vi "CRYPut To Curve Library.vi"(4 "O_Signal Type In":string[][](array[string]), 6 "I_Signal Type In":string[][](array[string]), 8 "O_Calibrated Device Name In":string[][](array[string]), 9 "I_Calibrated Device Name In":string[][](array[string]), 10 "Hardware In":string, 11 "Calibration Step Cluster":T3 {"Calibration 2D"."Sens Curve"."Z data" items=["dB", "Lin"]; "Calibration 2D"."Sens Curve"."X data" items=["dB", "Lin"]; "Calibration 2D"."Sens Curve"."Y data" items=["dB", "Lin"]; "Calibration 2D"."Sens Curve"."Z dB ref" format="%.1f"; "Calibration 2D"."Sens Curve"."Z axis" items=["Log", "Lin"]; "Calibration 2D"."Sens Curve"."X dB ref" format="%.1f"; "Calibration 2D"."Sens Curve"."X axis" items=["Log", "Lin"]; "Calibration 2D"."Sens Curve"."Y axis" items=["Log", "Lin"]; "Calibration 2D"."Sens Curve"."Y dB ref" format="%.1f"; "Calibration 2D"."Sens Curve"."Curve"."z" format="%.2f"; "Calibration 2D"."Sens Curve"."Curve"."y" format="%.2f"; "Calibration 2D"."Sens Curve"."Curve"."x" format="%.2f"; "Calibration 2D"."EQ Curve"."Z data" items=["dB", "Lin"]; "Calibration 2D"."EQ Curve"."X data" items=["dB", "Lin"]; "Calibration 2D"."EQ Curve"."Y data" items=["dB", "Lin"]; "Calibration 2D"."EQ Curve"."Z dB ref" format="%.1f"; "Calibration 2D"."EQ Curve"."Z axis" items=["Log", "Lin"]; "Calibration 2D"."EQ Curve"."X dB ref" format="%.1f"; "Calibration 2D"."EQ Curve"."X axis" items=["Log", "Lin"]; "Calibration 2D"."EQ Curve"."Y axis" items=["Log", "Lin"]; "Calibration 2D"."EQ Curve"."Y dB ref" format="%.1f"; "Calibration 2D"."EQ Curve"."Curve"."z" format="%.2f"; "Calibration 2D"."EQ Curve"."Curve"."y" format="%.2f"; "Calibration 2D"."EQ Curve"."Curve"."x" format="%.2f"; "Calibration 2D"."Corr Curve"."Z data" items=["dB", "Lin"]; "Calibration 2D"."Corr Curve"."X data" items=["dB", "Lin"]; "Calibration 2D"."Corr Curve"."Y data" items=["dB", "Lin"]; "Calibration 2D"."Corr Curve"."Z dB ref" format="%.1f"; "Calibration 2D"."Corr Curve"."Z axis" items=["Log", "Lin"]; "Calibration 2D"."Corr Curve"."X dB ref" format="%.1f"; "Calibration 2D"."Corr Curve"."X axis" items=["Log", "Lin"]; "Calibration 2D"."Corr Curve"."Y axis" items=["Log", "Lin"]; "Calibration 2D"."Corr Curve"."Y dB ref" format="%.1f"; "Calibration 2D"."Corr Curve"."Curve"."z" format="%.2f"; "Calibration 2D"."Corr Curve"."Curve"."y" format="%.2f"; "Calibration 2D"."Corr Curve"."Curve"."x" format="%.2f"; "Calibration 2D"."Calibration"."EQ Step size" items=["R10", "R20", "R40", "R80", "User"]; "Calibration 2D"."Calibration"."Corr Step size" items=["R10", "R20", "R40", "R80", "User"]}) -> (3 "Calibration flattened":string)   [LabVIEW 2013]
uses:
  Typedef Control/CRYCalibration All Cluster.ctl
  Typedef Control/CRYCalibration 2DCluster.ctl
  Typedef Control/CRYCalibration Cluster.ctl
  Typedef Control/CRYData Cluster.ctl
  Typedef Control/CRYData Cluster Array.ctl
  CRYProject/CRYProject Editor Global.vi
panel:
  out "Array":string[](array[string])
  out "Curve State":string[][](array[string])
  out "Values":T1 {"Z data" items=["dB", "Lin"]; "X data" items=["dB", "Lin"]; "Y data" items=["dB", "Lin"]; "Z dB ref" format="%.1f"; "Z axis" items=["Log", "Lin"]; "X dB ref" format="%.1f"; "X axis" items=["Log", "Lin"]; "Y axis" items=["Log", "Lin"]; "Y dB ref" format="%.1f"; "Curve"."z" format="%.2f"; "Curve"."y" format="%.2f"; "Curve"."x" format="%.2f"}
  out "Curve array":T1 {"Z data" items=["dB", "Lin"]; "X data" items=["dB", "Lin"]; "Y data" items=["dB", "Lin"]; "Z dB ref" format="%.1f"; "Z axis" items=["Log", "Lin"]; "X dB ref" format="%.1f"; "X axis" items=["Log", "Lin"]; "Y axis" items=["Log", "Lin"]; "Y dB ref" format="%.1f"; "Curve"."z" format="%.2f"; "Curve"."y" format="%.2f"; "Curve"."x" format="%.2f"}
  # "Insert Calibration curve and value into Curves Library"
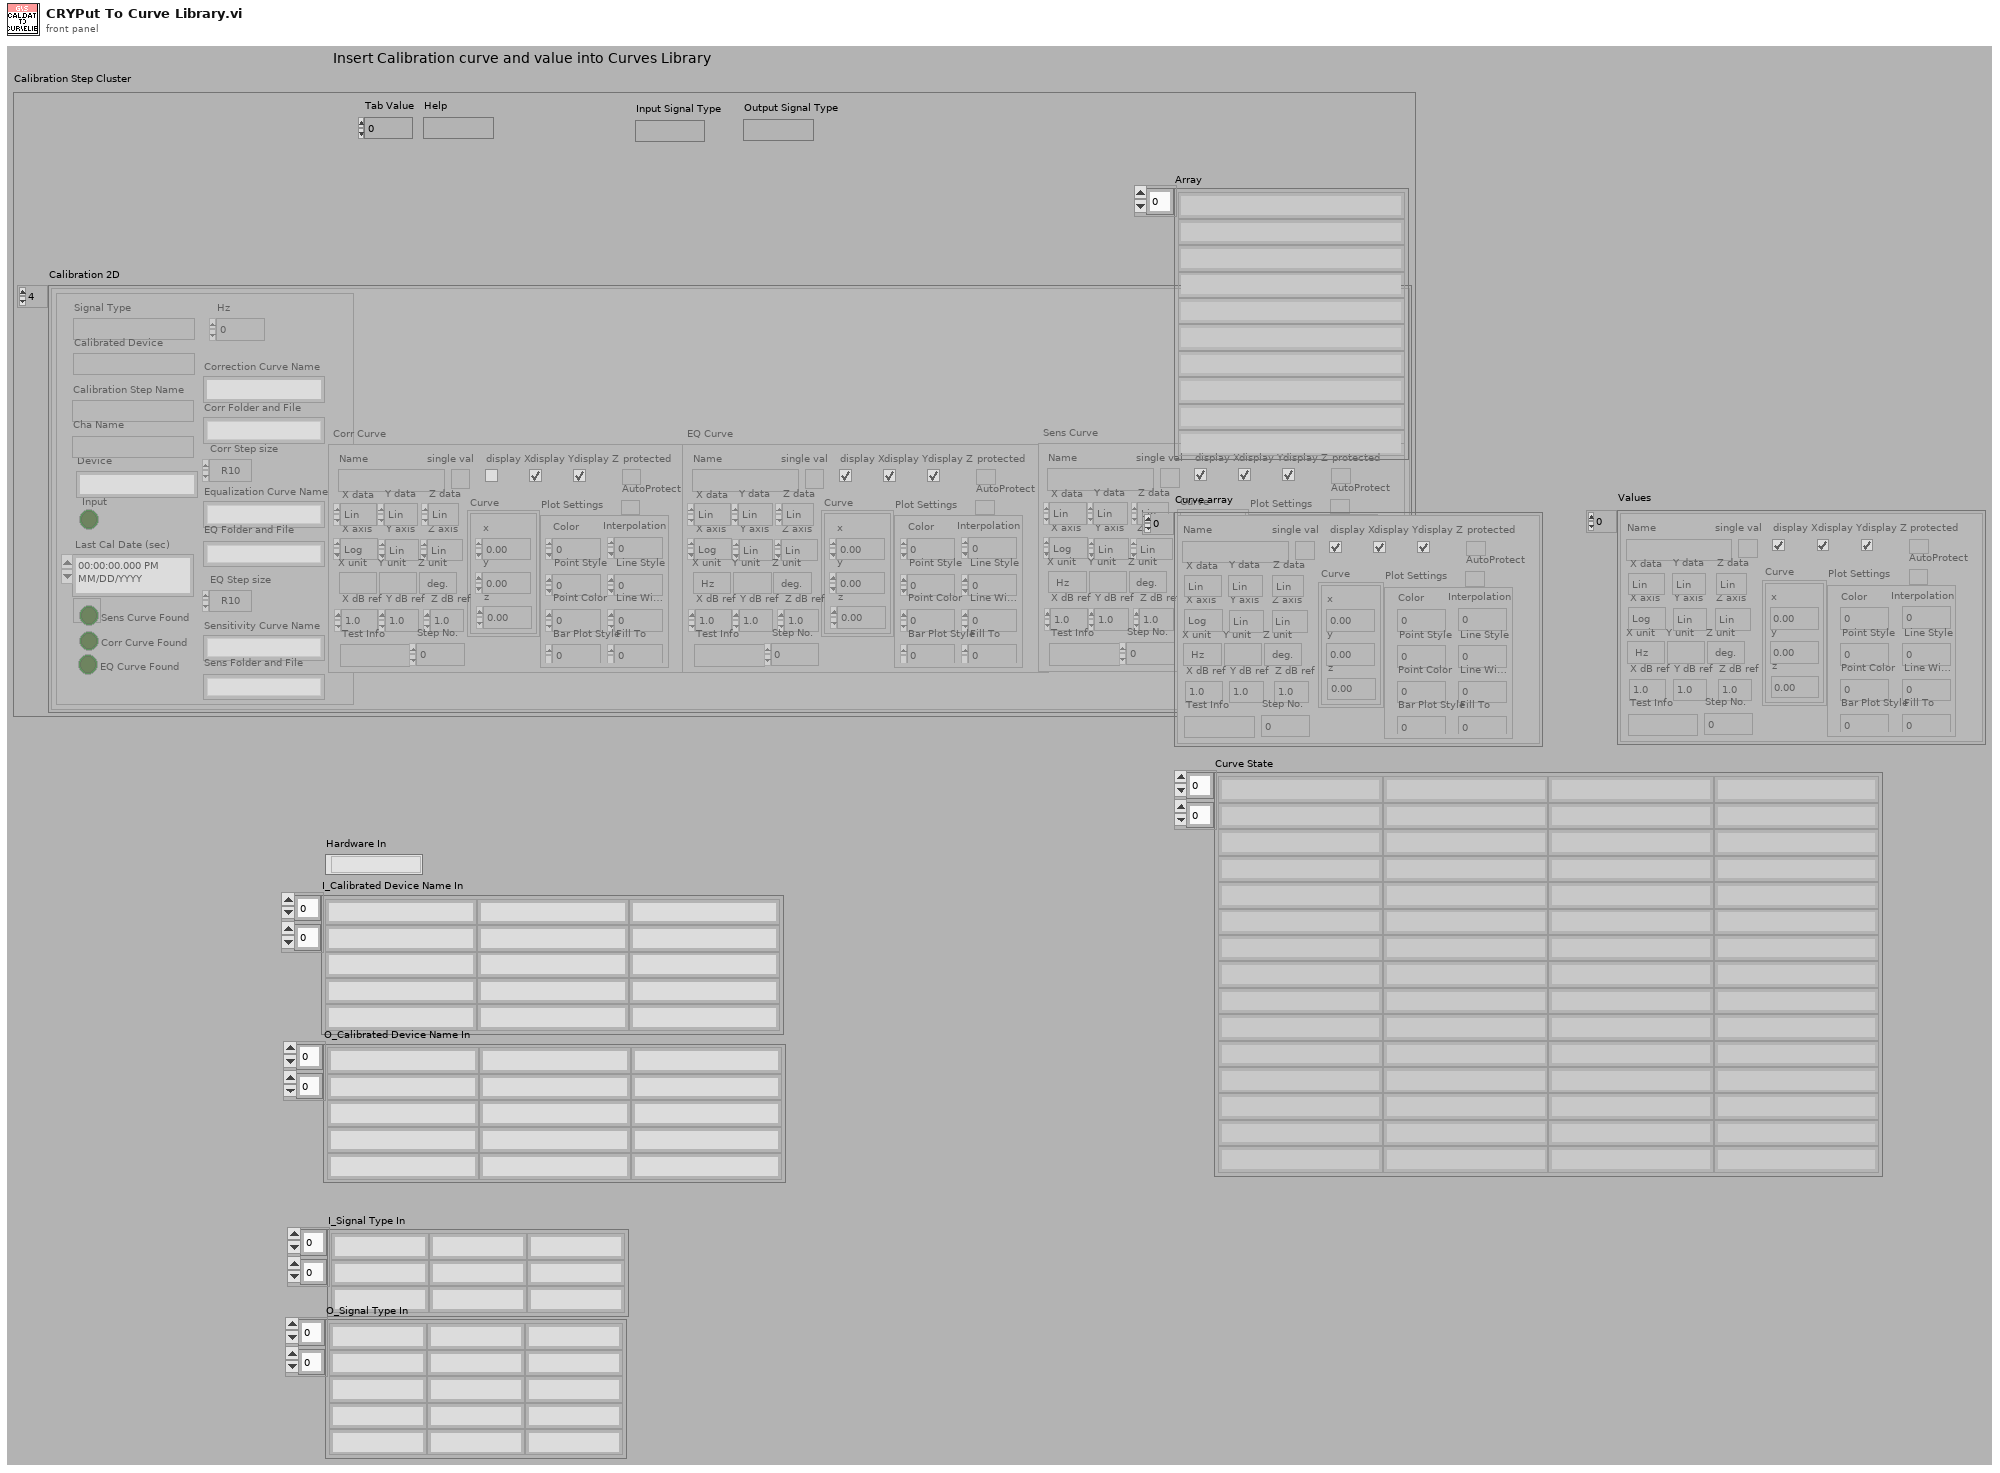
[diagram p1: front panel]
types:
  T1 = typedef "CRYData Cluster Array.ctl" = T2[]
  T2 = typedef "CRYData Cluster.ctl" = cluster{"Name":string, "Curve":cluster{"x":dbl, "y":dbl, "z":dbl}[], "X data":u16, "Y data":u16, "Z data":u16, "X axis":u16, "Y axis":u16, "Z axis":u16, "X unit":string, "Y unit":string, "Z unit":string, "X dB ref":dbl, "Y dB ref":dbl, "Z dB ref":dbl, "single val":bool, "protected":bool, "display X":bool, "display Y":bool, "display Z":bool, "Test Info":string, "Step No.":i32, "Plot Settings":cluster{"Color":u32, "Interpolation":u8, "Point Style":u8, "Line Style":u8, "Point Color":u32, "Line Width":u8, "Bar Plot Style":u8, "Fill To":i16}, "AutoProtect":bool}
  T3 = typedef "CRYCalibration All Cluster.ctl" = cluster{"Calibration 2D":T4[], "Help":string, "Tab Value":i32, "Input Signal Type":string, "Output Signal Type":string}
  T4 = typedef "CRYCalibration 2DCluster.ctl" = cluster{"Calibration":T5, "Corr Curve":T2, "EQ Curve":T2, "Sens Curve":T2}
  T5 = typedef "CRYCalibration Cluster.ctl" = cluster{"Calibration Step Name":string, "Device":string, "Correction Curve Name":string, "Equalization Curve Name":string, "Sensitivity Curve Name":string, "Corr Folder and File":string, "EQ Folder and File":string, "Sens Folder and File":string, "Corr Step size":u16, "EQ Step size":u16, "Input":bool, "Last Cal Date (sec)":timestamp, "Cha Name":string, "Corr Curve Found":bool, "EQ Curve Found":bool, "Sens Curve Found":bool, "Signal Type":string, "Calibrated Device":string, "Hz":u32}
  T6 = typedef "CRYChanged Names Cluster.ctl" = cluster{"Input Channel":T7, "Output Channel":T7, "Cuve":T7, "Value":T7, "Result":T7, "Wave":T7}
  T7 = typedef "CRYChanged Data Array Cluster.ctl" = cluster{"Rename":T8[], "Delete":T8[]}
  T8 = typedef "CRYChanged Data Cluster.ctl" = cluster{"Old Name":string, "New Name":string}
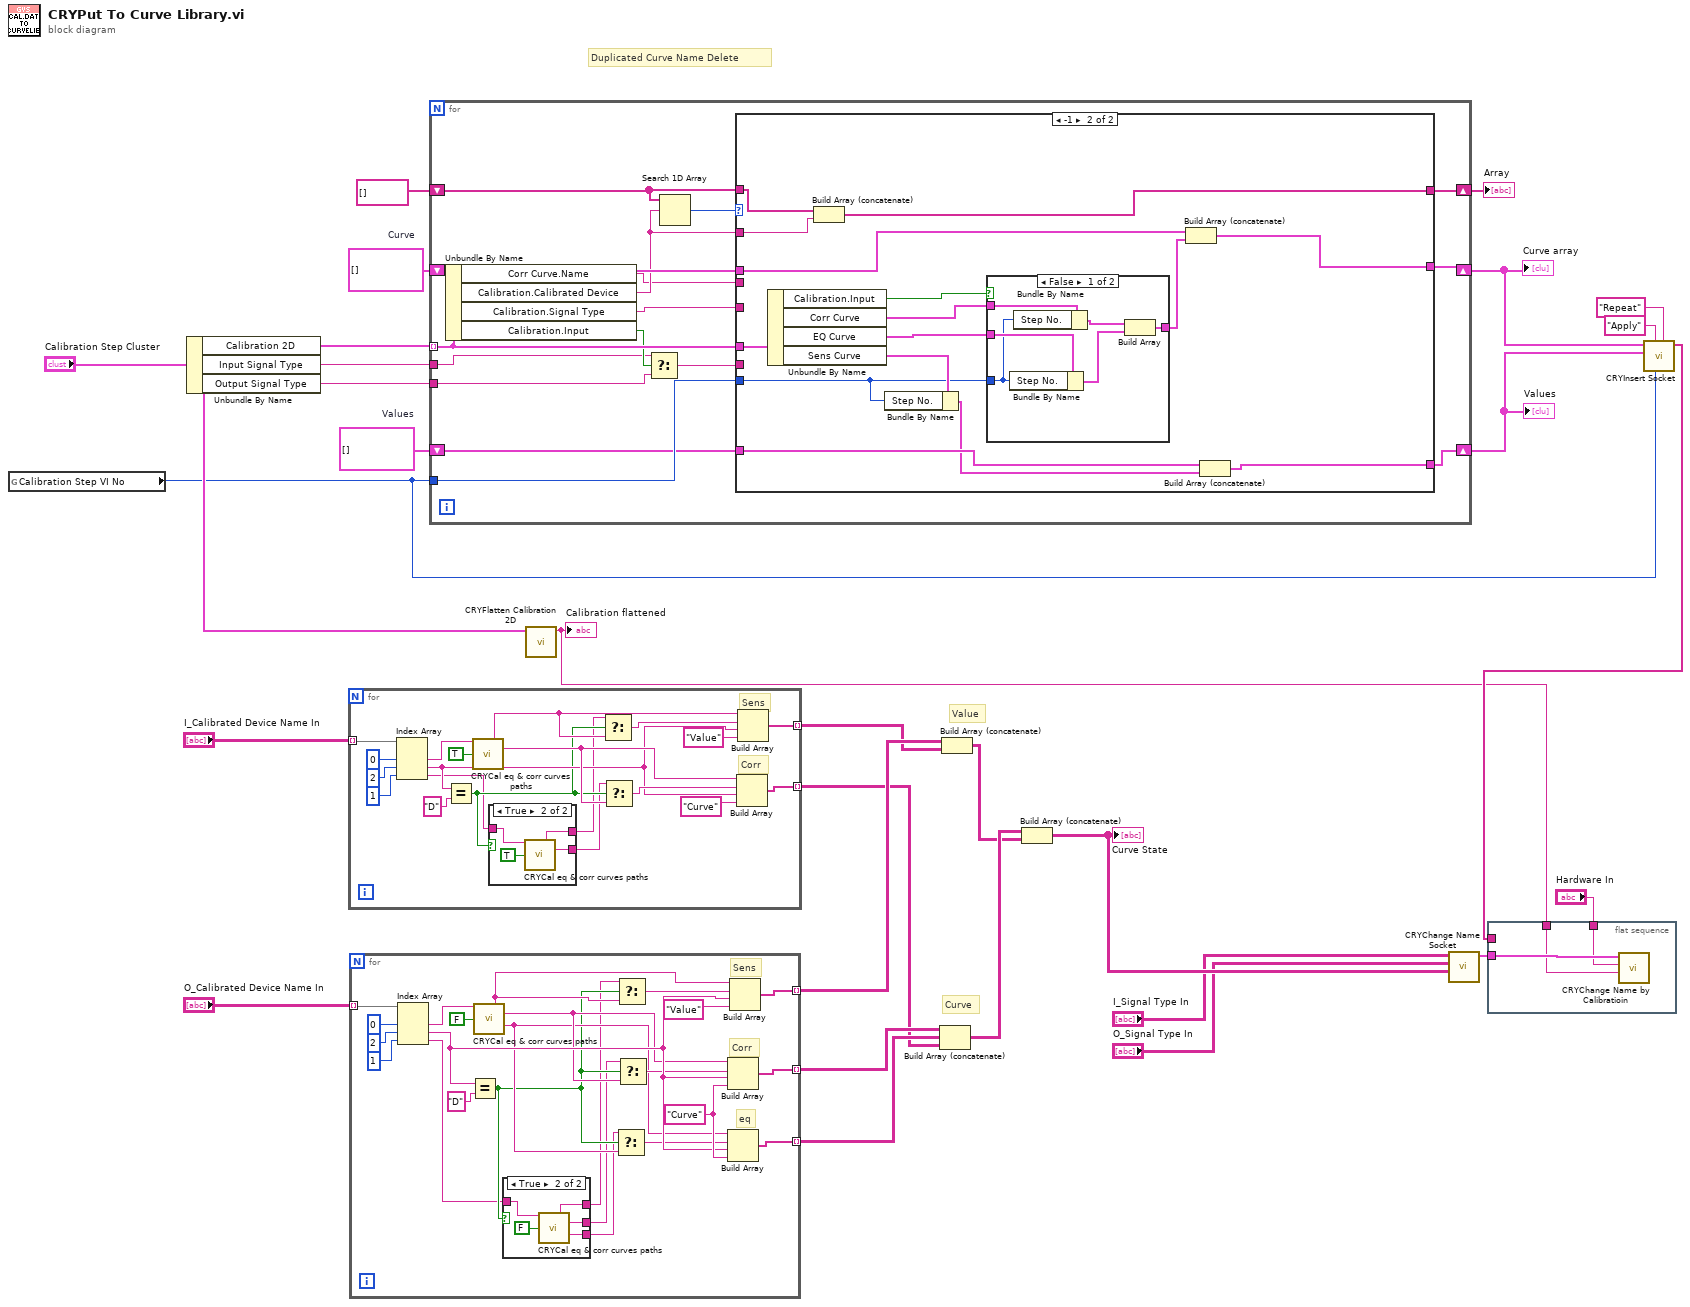
[diagram p0: block diagram]
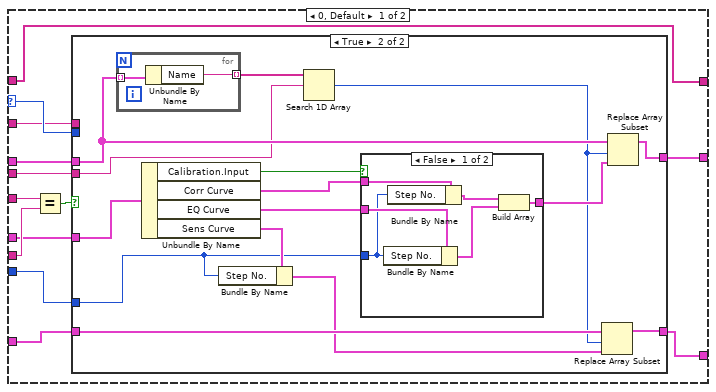
[diagram p4: hidden frame]
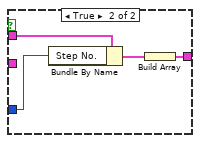
[diagram p6: hidden frame]
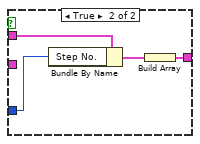
[diagram p7: hidden frame]
diagram:
  w21 = T1 []  # Values
  w25 = T1 []  # Curve
  # "Curve"
  # "Value"
  # "Duplicated Curve Name Delete"
  n1 = global read "CRYProject Editor Global.vi" "Calibration Step VI No"() -> (w24:i32)
  n2 = Unbundle By Name("Calibration Step Cluster") -> ("Calibration 2D"=w27:T4[], "Input Signal Type"=w3:string, "Output Signal Type"=w2:string)
  n3 = for {
    tunnel: "I_Calibrated Device Name In" -> [w49] mode=indexing
    tunnel: [w44] -> w16 mode=indexing
    tunnel: [w43] -> w13 mode=indexing
    # "Corr"
    # "Sens"
    n4 = Index Array(array=w49, index #1=0 ("index"), index #2=2 ("index"), index #3=1 ("index")) -> (element #1=w48:string, element #2=w36:string, element #3=w32:string)
    n5 = Equal?(x=w36, y="D" ("element")) -> (x = y?=w33:bool)
    n6 = call "CRYCal eq & corr curves paths.vi"("Calibrated Device Name"=w48, "In_Out"=TRUE) -> ("Sens Currve Name"=w35:string, "Corr Curve Name"=w39:string)  [unwired: 1 in, 11 out]
    n7 = case shown="True" w33 {
      tunnel: w32 -> [_ w52]
      tunnel: [_ w51] -> w31
      tunnel: [_ w50] -> w30
      frame False {
      }
      frame True {
        n8 = call "CRYCal eq & corr curves paths.vi"("Calibrated Device Name"=w52, "In_Out"=TRUE) -> ("Sens Currve Name"=w51:string, "Corr Curve Name"=w50:string)  [unwired: 1 in, 11 out]
      }
    }
    n9 = Select(t=w31, s=w33, f=w35) -> (s? t:f=w34:string)
    n10 = Select(t=w30, s=w33, f=w39) -> (s? t:f=w37:string)
    n11 = Build Array(w39, w37, w36, "Curve" ("element")) -> (w43:string[])
    n12 = Build Array(w35, w34, w36, "Value" ("element")) -> (w44:string[])
  }
  n13 = for {
    tunnel: "O_Calibrated Device Name In" -> [w77] mode=indexing
    tunnel: [w72] -> w17 mode=indexing
    tunnel: [w71] -> w15 mode=indexing
    tunnel: [w70] -> w14 mode=indexing
    w69 = "Curve" ("element")
    # "eq"
    # "Corr"
    # "Sens"
    n14 = Index Array(array=w77, index #1=0 ("index"), index #2=2 ("index"), index #3=1 ("index")) -> (element #1=w76:string, element #2=w66:string, element #3=w57:string)
    n15 = Equal?(x=w66, y="D" ("element")) -> (x = y?=w58:bool)
    n16 = call "CRYCal eq & corr curves paths.vi"("Calibrated Device Name"=w76, "In_Out"=FALSE) -> ("Sens Currve Name"=w62:string, "Corr Curve Name"=w64:string, "EQ Curve Name"=w60:string)  [unwired: 1 in, 10 out]
    n17 = case shown="True" w58 {
      tunnel: w57 -> [_ w81]
      tunnel: [_ w80] -> w54
      tunnel: [_ w79] -> w55
      tunnel: [_ w78] -> w56
      frame False {
      }
      frame True {
        n18 = call "CRYCal eq & corr curves paths.vi"("Calibrated Device Name"=w81, "In_Out"=FALSE) -> ("Sens Currve Name"=w80:string, "Corr Curve Name"=w79:string, "EQ Curve Name"=w78:string)  [unwired: 1 in, 10 out]
      }
    }
    n19 = Select(t=w56, s=w58, f=w60) -> (s? t:f=w59:string)
    n20 = Select(t=w54, s=w58, f=w62) -> (s? t:f=w61:string)
    n21 = Select(t=w55, s=w58, f=w64) -> (s? t:f=w63:string)
    n22 = Build Array(w64, w63, w66, w69) -> (w71:string[])
    n23 = Build Array(w60, w59, w66, w69) -> (w70:string[])
    n24 = Build Array(w62, w61, w66, "Value" ("element")) -> (w72:string[])
  }
  n25 = for {
    tunnel: w27 -> [w91] mode=indexing
    shift-right: [w94] -> w29
    shift-left: w25 -> [w95]
    tunnel: w24 -> [w90]
    shift-right: [w96] -> w1
    shift-left: string[] [] ("Array") -> [w97]
    shift-right: [w92] -> w20
    shift-left: w21 -> [w89]
    tunnel: w3 -> [w87]
    tunnel: w2 -> [w86]
    n26 = Unbundle By Name(w91) -> ("Corr Curve.Name"=w83:string, "Calibration.Calibrated Device"=w93:string, "Calibration.Signal Type"=w85:string, "Calibration.Input"=w88:bool)
    n27 = Select(t=w87, s=w88, f=w86) -> (s? t:f=w84:string)
    n28 = Search 1D Array(1D array=w97, element=w93) -> (index of element=w98:i32)  [unwired: 1 in]
    n29 = case shown="-1" w98 {
      selector: w98 -> [w103 _]
      tunnel: w93 -> [w100 w155]
      tunnel: w97 -> [w107 w154]
      tunnel: [w107 w153] -> w96
      tunnel: w95 -> [w110 w152]
      tunnel: [w111 w151] -> w94
      tunnel: [w104 w144] -> w92
      tunnel: w91 -> [w102 w146]
      tunnel: w90 -> [w106 w145]
      tunnel: w89 -> [w105 w143]
      tunnel: w85 -> [w101 _]
      tunnel: w84 -> [w109 _]
      tunnel: w83 -> [w99 _]
      frame 0, Default {
        n30 = Equal?(x=w101, y=w109) -> (x = y?=w108:bool)
        n31 = case shown="True" w108 {
          tunnel: [w113 w124] -> w111
          tunnel: w110 -> [w113 w117]
          tunnel: w106 -> [_ w122]
          tunnel: w105 -> [w112 w121]
          tunnel: [w112 w120] -> w104
          tunnel: w103 -> [_ _]
          tunnel: w102 -> [_ w118]
          tunnel: w100 -> [_ _]
          tunnel: w99 -> [_ w114]
          frame False {
          }
          frame True {
            n32 = for {
              tunnel: w117 -> [w130] mode=indexing
              tunnel: [w129] -> w116 mode=indexing
              n33 = Unbundle By Name(w130) -> ("Name"=w129:string)
            }
            n34 = Unbundle By Name(w118) -> ("Calibration.Input"=w128:bool, "Corr Curve"=w126:T2, "EQ Curve"=w127:T2, "Sens Curve"=w125:T2)
            n35 = Bundle By Name(cluster=w125, "Step No."=w122) -> (w119:T2)
            n36 = Search 1D Array(1D array=w116, element=w114) -> (index of element=w115:i32)  [unwired: 1 in]
            n37 = case shown="False" w128 {
              tunnel: w127 -> [w135 _]
              tunnel: w126 -> [w134 w139]
              tunnel: [w136 w140] -> w123
              tunnel: w122 -> [w131 w137]
              frame False {
                n38 = Bundle By Name(cluster=w135, "Step No."=w131) -> (w133:T2)
                n39 = Bundle By Name(cluster=w134, "Step No."=w131) -> (w132:T2)
                n40 = Build Array(w132, w133) -> (w136:T2[])
              }
              frame True {
                n41 = Bundle By Name(cluster=w139, "Step No."=w137) -> (w138:T2)
                n42 = Build Array(w138) -> (w140:T2[])
              }
            }
            n43 = Replace Array Subset(array=w121, new element=w119, index=w115) -> (w120:T1)
            n44 = Replace Array Subset(array=w117, new element=w123, index=w115) -> (w124:T1)
          }
        }
      }
      frame -1 {
        n45 = Unbundle By Name(w146) -> ("Calibration.Input"=w150:bool, "Corr Curve"=w148:T2, "EQ Curve"=w149:T2, "Sens Curve"=w147:T2)
        n46 = Build Array (concatenate)(w154, w155) -> (w153:string[])
        n47 = Bundle By Name(cluster=w147, "Step No."=w145) -> (w142:T2)
        n48 = case shown="False" w150 {
          tunnel: w149 -> [w160 _]
          tunnel: w148 -> [w159 w164]
          tunnel: [w161 w165] -> w141
          tunnel: w145 -> [w156 w162]
          frame False {
            n49 = Bundle By Name(cluster=w160, "Step No."=w156) -> (w158:T2)
            n50 = Bundle By Name(cluster=w159, "Step No."=w156) -> (w157:T2)
            n51 = Build Array(w157, w158) -> (w161:T2[])
          }
          frame True {
            n52 = Bundle By Name(cluster=w164, "Step No."=w162) -> (w163:T2)
            n53 = Build Array(w163) -> (w165:T2[])
          }
        }
        n54 = Build Array (concatenate)(w152, w141) -> (w151:T1)
        n55 = Build Array (concatenate)(w143, w142) -> (w144:T1)
      }
    }
  }
  "Curve array" <- w29
  "Values" <- w20
  "Array" <- w1
  n56 = call "CRYFlatten Calibration 2D.vi"("Calibration All Cluster"="Calibration Step Cluster") -> ("Calibration flattened"=w7:string)  [unwired: 10 out]
  "Calibration flattened" <- w7
  n57 = Build Array (concatenate)(w15, w14, w13) -> (w12:string[][])
  n58 = Build Array (concatenate)(w17, w16) -> (w11:string[][])
  n59 = Build Array (concatenate)(w12, w11) -> (w6:string[][])
  "Curve State" <- w6
  n60 = call "CRYChange Name Socket.vi"("Data"=w6, "O_Signal Type"="O_Signal Type In", "I_Signal Type"="I_Signal Type In") -> ("Changed Name"=w10:T6)  [unwired: 8 in]
  n61 = flat-sequence {
    tunnel: w10 -> [w168]
    tunnel: w7 -> [w166]
    tunnel: "Hardware In" -> [w167]
    tunnel: w8 -> [_]
    frame #0 {
      n62 = call "CRYChange Name by Calibratioin.vi"("Calibration In"=w166, "Hardware In"=w167, "Changed Names"=w168) -> ()  [unwired: 9 in]
    }
  }
  n63 = call "CRYInsert Socket.vi"("sOption2"="Repeat", "Step No."=w24, "sOption1"="Apply" ("sOption"), "Values"=w20, "Curves"=w29) -> ("Inserted Names Out"=w8:string[])  [unwired: 6 in]
